vi "Get Water Level.vi"(8 "error in (no error)":errorcluster, 11 "Simulated Water Level in":refnum<class "Simulated Water Level.lvclass">) -> (0 "error out":errorcluster, 2 "Water Level":dbl)   [LabVIEW 2025, in "Simulated Water Level.lvclass"]
uses:
  Simulated Water Level.lvclass
  Cooler Plug-Ins/Simulated Evaporative Cooler.lvclass/Simulation Data_Global.vi
  Cooler Plug-Ins/Simulated Evaporative Cooler.lvclass/Simulated Evaporative Cooler.lvclass
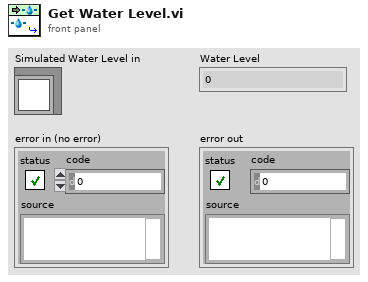
[diagram p1: front panel]
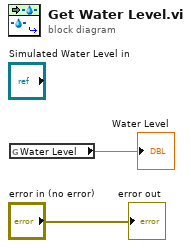
[diagram p0: block diagram]
diagram:
  n1 = global read "Simulation Data_Global.vi" "Water Level"() -> (→"Water Level":dbl)
  "error out" <- "error in (no error)"
